vi "Read Show.vi"(8 "error in (no error)":errorcluster, 11 "FSM.Annotation in":refnum<class "FSM.Annotation.lvclass">) -> (0 "error out":errorcluster, 2 "Show":bool, 3 "FSM.Annotation out":refnum<class "FSM.Annotation.lvclass">)   [LabVIEW 2020, in "FSM.Annotation.lvclass"]
uses:
  FSM.Annotation.lvclass
  FSM.Annotation.lvclass/FSM.Annotation.ctl
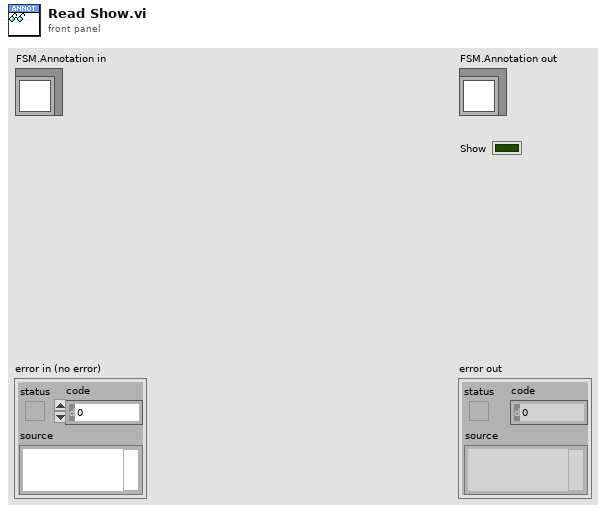
[diagram p1: front panel]
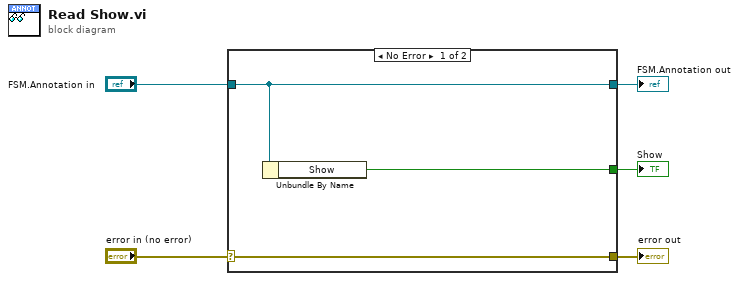
[diagram p0: block diagram]
diagram:
  n1 = case shown="No Error" "error in (no error)" {
    selector: "error in (no error)" -> [w8 w9]
    tunnel: [w8 w9] -> w4
    tunnel: [w7 w10] -> w2
    tunnel: "FSM.Annotation in" -> [w7 w10]
    tunnel: [w6 _] -> w1
    frame No Error {
      n2 = Unbundle By Name(w7) -> ("Show"=w6:bool)
    }
    frame Error {
    }
  }
  "error out" <- w4
  "FSM.Annotation out" <- w2
  "Show" <- w1
